vi "Refine triangles, centroid recursive.vi"(0 "Original STL file path":path=path "C:/EnFlo Software/Anemometry/Utilities/Probe blockage potential flow sim/test stl files/Sphere.stl", 1 "Refined STL file path":path, 2 "Refinement stages":u8=1, 3 "Refinement point":u8(ring) items=["Centroid", "Barycenter", "Random"], 4 "Write STL file":bool) -> (5 "N triangles before refinement":i32, 6 "N triangles after refinement":i32)   [LabVIEW 2017]
uses:
  <vilib>/Utility/miscctls.llb/LVRGBAColorTypeDef.ctl
  ctls/Triangle panel.ctl
panel:
  in  "Render mode":T1(ring)=enum."Wireframe"
  out "Refined STL view":refnum<vi>(3d-picture)
  out "Original STL view":refnum<vi>(3d-picture)
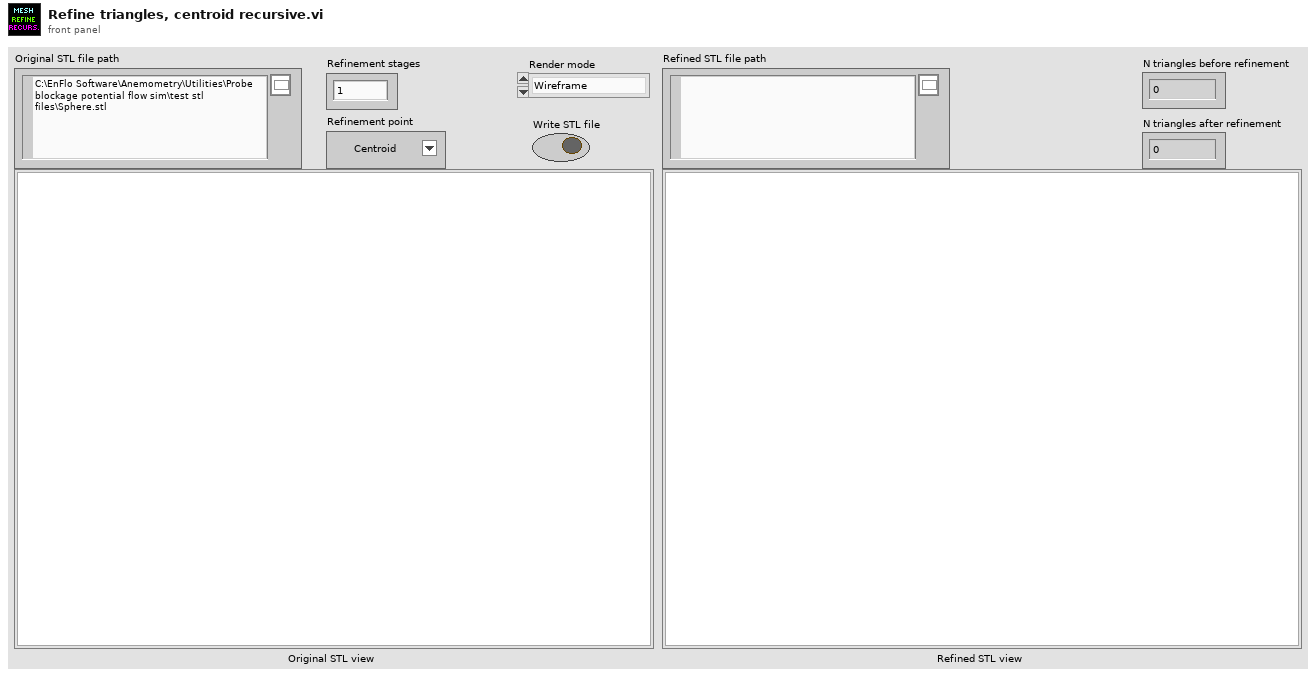
[diagram p1: front panel]
types:
  T1 = enum16{"Inherit Value", "Points", "Wireframe", "Polygons"}
  T2 = typedef "Triangle panel.ctl" = cluster{"V0":sgl[], "V1":sgl[], "V2":sgl[], "E0":sgl[], "E1":sgl[], "E2":sgl[], "n^":sgl[], "Pc":sgl[], "Gamma'":sgl, "V_transp.":sgl, "E0 link":i32, "E1 link":i32, "E2 link":i32}
  T3 = typedef "LVRGBAColorTypeDef.ctl" = cluster{"Red":sgl, "Green":sgl, "Blue":sgl, "Alpha":sgl}
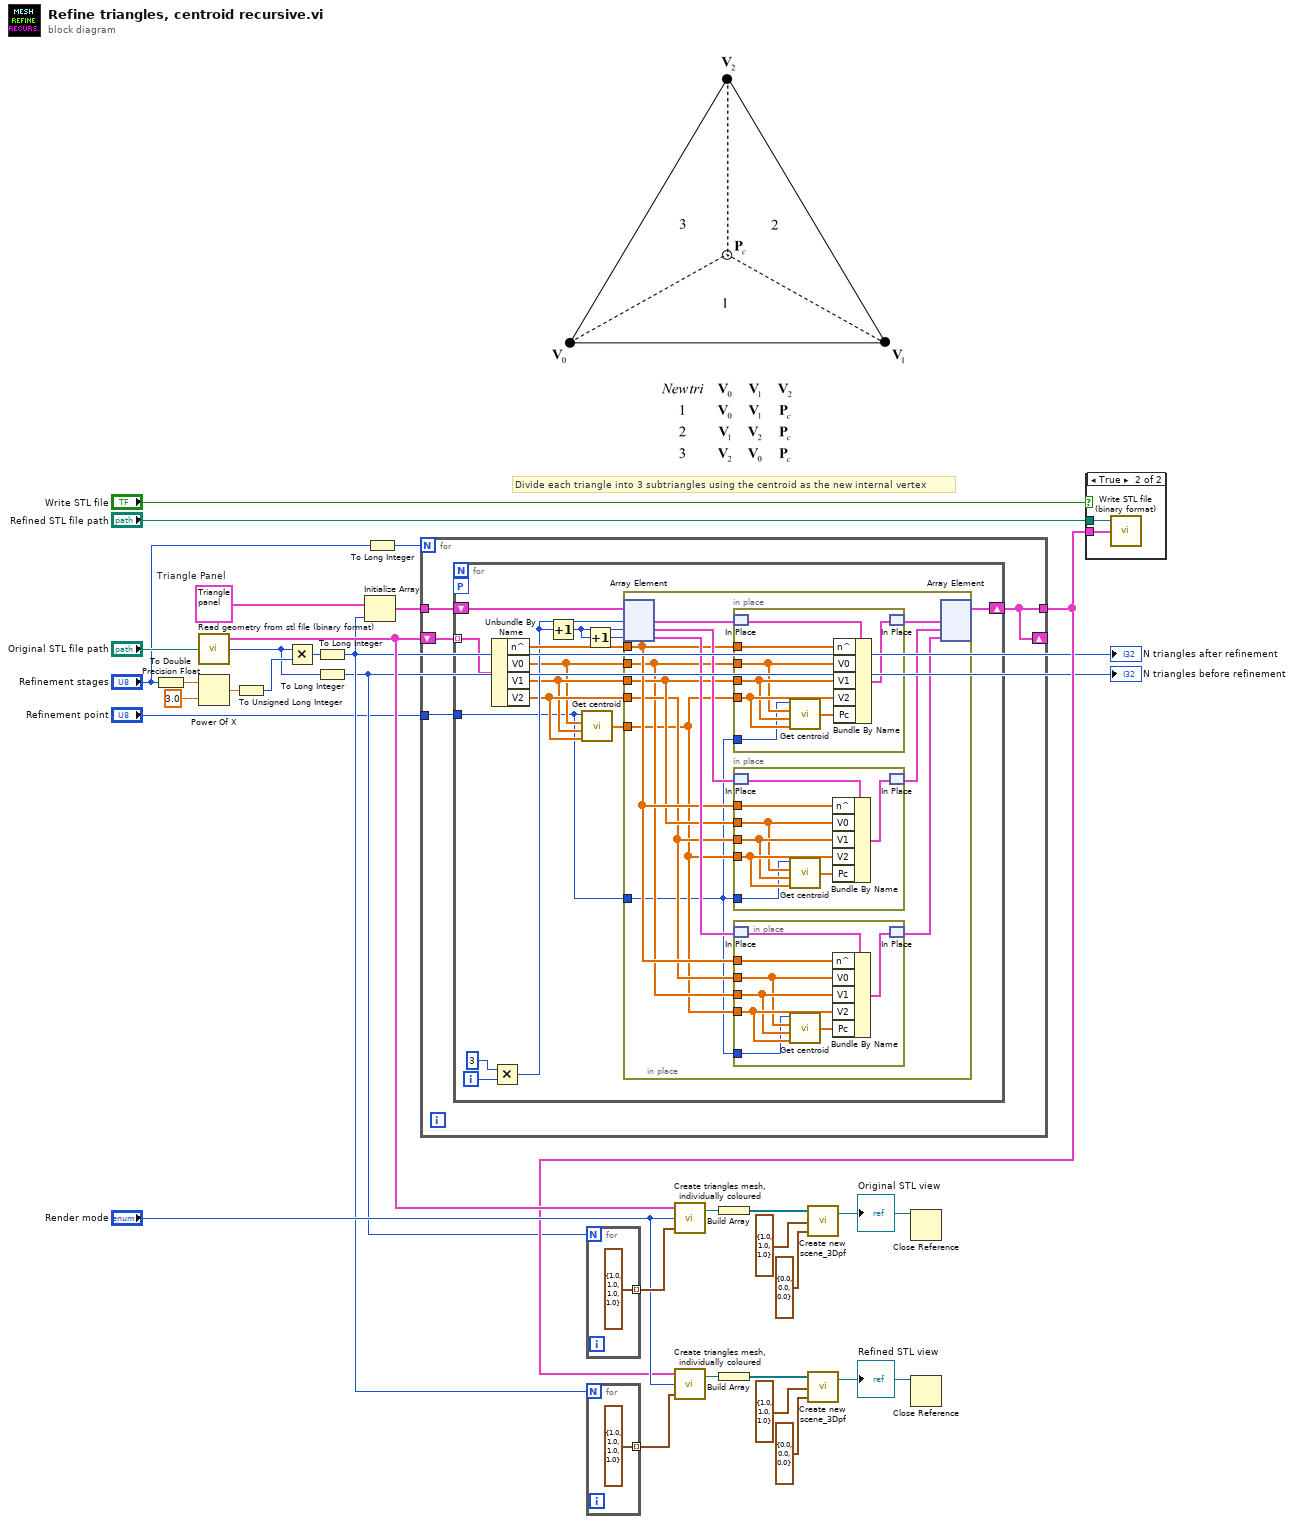
[diagram p0: block diagram]
diagram:
  w31 = T2 {"V0"=[], "V1"=[], "V2"=[], "E0"=[], "E1"=[], "E2"=[], "n^"=[], "Pc"=[], "Gamma'"=0.0, "V_transp."=0.0, "E0 link"=-1, "E1 link"=-1, "E2 link"=-1}  # Triangle Panel
  # "Divide each triangle into 3 subtriangles using the centroid as the new internal vertex"
  n1 = To Double Precision Float(number="Refinement stages") -> (double precision float=w21:dbl)
  n2 = call "Read geometry from stl file (binary format).vi"("STL file path"="Original STL file path") -> ("Panel triangles array"=w15:T2[], "N triangles"=w13:u32)  [unwired: 1 out]
  n3 = Power Of X(1:3.0 ("x"), 2:w21) -> (0:w24:dbl)
  n4 = To Unsigned Long Integer(number=w24) -> (unsigned 32bit integer=w22:u32)
  n5 = Multiply(x=w13, y=w22) -> (x*y=w23:u32)
  n6 = To Long Integer(number=w23) -> (32bit integer=w6:i32)
  "N triangles after refinement" <- w6
  n7 = To Long Integer(number=w13) -> (32bit integer=w3:i32)
  "N triangles before refinement" <- w3
  n8 = Initialize Array(w31, w6) -> (w16:T2[])
  n9 = To Long Integer(number="Refinement stages") -> (32bit integer=w4:i32)
  n10 = for {
    N: w4 -> [_]
    tunnel: w16 -> [w35]
    tunnel: [w33] -> w14
    shift-right: [w33] -> _
    shift-left: w15 -> [w34]
    tunnel: "Refinement point" -> [w32]
    n11 = for {
      tunnel: w34 -> [w46] mode=indexing
      shift-right: [w44] -> w33
      shift-left: w35 -> [w47]
      workers-P: _ -> [_]
      tunnel: w32 -> [w36]
      i -> [w49]
      n12 = Unbundle By Name(w46) -> ("n^"=w45:sgl[], "V0"=w37:sgl[], "V1"=w38:sgl[], "V2"=w39:sgl[])
      n13 = Multiply(x=3, y=w49) -> (x*y=w43:i32)
      n14 = Increment(x=w43) -> (x+1=w42:i32)
      n15 = call "Get centroid.vi"("V2"=w39, "V1"=w38, "V0"=w37, "Centroid type"=w36) -> ("Pc"=w40:sgl[])
      n16 = Increment(x=w42) -> (x+1=w41:i32)
      n17 = in-place {
        in-place-border: w45 -> [w55]
        in-place-border: w37 -> [w52]
        in-place-border: w38 -> [w54]
        in-place-border: w40 -> [w51]
        in-place-border: w39 -> [w53]
        in-place-border: w36 -> [w50]
        n18 = in-place-array #1(w47, w43, w42, w41) -> (w61:T2, w59:T2, w58:T2)
        n19 = in-place {
          in-place-border: w55 -> [w67]
          in-place-border: w52 -> [w64]
          in-place-border: w54 -> [w65]
          in-place-border: w51 -> [w66]
          in-place-border: w50 -> [w63]
          n20 = in-place-match #2(w61) -> (w69:T2)
          n21 = call "Get centroid.vi"("V2"=w66, "V1"=w65, "V0"=w64, "Centroid type"=w63) -> ("Pc"=w62:sgl[])
          n22 = Bundle By Name(cluster=w69, "n^"=w67, "V0"=w64, "V1"=w65, "V2"=w66, "Pc"=w62) -> (w68:T2)
          n23 = in-place-match #2(w68) -> (w60:T2)
        }
        n24 = in-place {
          in-place-border: w55 -> [w75]
          in-place-border: w54 -> [w71]
          in-place-border: w53 -> [w72]
          in-place-border: w51 -> [w73]
          in-place-border: w50 -> [w70]
          n25 = in-place-match #3(w59) -> (w77:T2)
          n26 = call "Get centroid.vi"("V2"=w73, "V1"=w72, "V0"=w71, "Centroid type"=w70) -> ("Pc"=w74:sgl[])
          n27 = Bundle By Name(cluster=w77, "n^"=w75, "V0"=w71, "V1"=w72, "V2"=w73, "Pc"=w74) -> (w76:T2)
          n28 = in-place-match #3(w76) -> (w57:T2)
        }
        n29 = in-place {
          in-place-border: w55 -> [w83]
          in-place-border: w53 -> [w79]
          in-place-border: w52 -> [w80]
          in-place-border: w51 -> [w81]
          in-place-border: w50 -> [w78]
          n30 = in-place-match #4(w58) -> (w85:T2)
          n31 = call "Get centroid.vi"("V2"=w81, "V1"=w80, "V0"=w79, "Centroid type"=w78) -> ("Pc"=w82:sgl[])
          n32 = Bundle By Name(cluster=w85, "n^"=w83, "V0"=w79, "V1"=w80, "V2"=w81, "Pc"=w82) -> (w84:T2)
          n33 = in-place-match #4(w84) -> (w56:T2)
        }
        n34 = in-place-array #1(w60, w57, w56) -> (w44:T2[])  [unwired: 3 out]
      }
    }
  }
  n35 = for {
    N: w3 -> [_]
    tunnel: [T3 {"Red"=1.0, "Green"=1.0, "Blue"=1.0, "Alpha"=1.0} ("Colour")] -> w20 mode=indexing
  }
  n36 = for {
    N: w6 -> [_]
    tunnel: [T3 {"Red"=1.0, "Green"=1.0, "Blue"=1.0, "Alpha"=1.0} ("Colour")] -> w7 mode=indexing
  }
  n37 = call "Create triangles mesh, individually coloured.vi"("Colours array"=w20, "Render mode"="Render mode", "Triangles array"=w15) -> ("Triangle mesh out"=w28:refnum<vi>)  [unwired: 1 out]
  n38 = call "Create triangles mesh, individually coloured.vi"("Colours array"=w7, "Render mode"="Render mode", "Triangles array"=w14) -> ("Triangle mesh out"=w9:refnum<vi>)  [unwired: 1 out]
  n39 = Build Array(w28) -> (w29:refnum<vi>[])
  n40 = Build Array(w9) -> (w10:refnum<vi>[])
  n41 = call "Create new scene_3Dpf.vi"("Translation"=cluster{"X":sgl, "Y":sgl, "Z":sgl} {"X"=0.0, "Y"=0.0, "Z"=0.0}, "Scale"=cluster{"X":sgl, "Y":sgl, "Z":sgl} {"X"=1.0, "Y"=1.0, "Z"=1.0}, "Scene objects array"=w29) -> ("Scene out"=w30:refnum<vi>)  [unwired: 1 out]
  "Original STL view" <- w30
  n42 = call "Create new scene_3Dpf.vi"("Translation"=cluster{"X":sgl, "Y":sgl, "Z":sgl} {"X"=0.0, "Y"=0.0, "Z"=0.0}, "Scale"=cluster{"X":sgl, "Y":sgl, "Z":sgl} {"X"=1.0, "Y"=1.0, "Z"=1.0}, "Scene objects array"=w10) -> ("Scene out"=w8:refnum<vi>)  [unwired: 1 out]
  "Refined STL view" <- w8
  n43 = Close Reference(reference=w30) -> ()  [unwired: 1 in, 1 out]
  n44 = Close Reference(reference=w8) -> ()  [unwired: 1 in, 1 out]
  n45 = case shown="True" "Write STL file" {
    tunnel: "Refined STL file path" -> [_ w89]
    tunnel: w14 -> [_ w88]
    frame False {
    }
    frame True {
      n46 = call "Write STL file (binary format).vi"("Panel triangles array"=w88, "STL file path"=w89) -> ()  [unwired: 2 in, 1 out]
    }
  }
